vi "myRIO v1.0 Enable Encoder.vi"(8 "error in (no error)":errorcluster, 9 "Enable":bool, 10 "Channel":T1, 11 "myRIO Ref In":T2) -> (0 "error out":errorcluster, 3 "myRIO Ref Out":T2)   [LabVIEW 2021]
uses:
  <vilib>/myRIO/Common/Instrument Driver Framework/Utilities/typedefs/myRIO v1.0 Reference.ctl
  <vilib>/myRIO/Common/Instrument Driver Framework/Utilities/typedefs/Generic FPGA Reference.ctl
  <vilib>/myRIO/Common/Instrument Driver Framework/myRIO v1.0/Encoder/typedefs/Encoder Channels Enum.ctl
  <vilib>/myRIO/Common/Instrument Driver Framework/myRIO v1.0/Encoder/typedefs/Encoder Channels FPGA Reference.ctl
  <vilib>/rvi/errors/niLvFpgaAdjustHostInterfaceError.vi
  <vilib>/rvi/interface/nirviReadWriteControl/nirviReadWriteControl.xnode
  <vilib>/rvi/interface/Simulation/niFpgaSimulationCallBeginRW.vi
  NiFpgaLv.dll
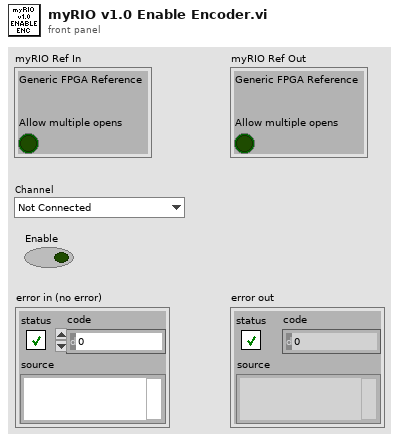
[diagram p1: front panel]
types:
  T1 = typedef "Encoder Channels Enum.ctl" = enum16{"Not Connected", "C/ENC0", "C/ENC1", "A/ENC", "A/ENC0", "A/ENC1", "A/ENC2", "A/ENC3", "A/ENC4", "A/ENC5", "A/ENC6", "A/ENC7", "A/ENC8", "A/ENC9", "B/ENC", "B/ENC0", "B/ENC1", "B/ENC2", "B/ENC3", "B/ENC4", "B/ENC5", "B/ENC6", "B/ENC7", "B/ENC8", "B/ENC9", "DIO/ENC0", "DIO/ENC1", "DIO/ENC2", "DIO/ENC3", "DIO/ENC4"}
  T2 = typedef "myRIO v1.0 Reference.ctl" = cluster{"Generic FPGA Reference":T3, "Allow multiple opens":bool}
  T3 = typedef "Generic FPGA Reference.ctl" = refnum<k20>
  T4 = typedef "Encoder Channels FPGA Reference.ctl" = refnum<k20>
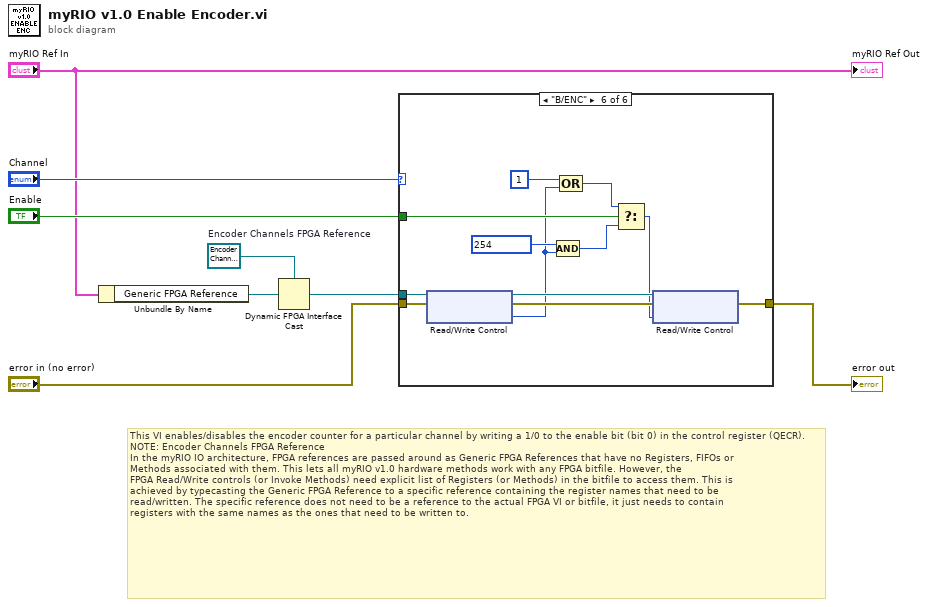
[diagram p0: block diagram]
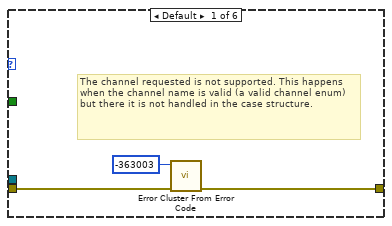
[diagram p2: hidden frame]
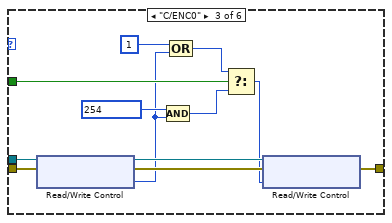
[diagram p4: hidden frame]
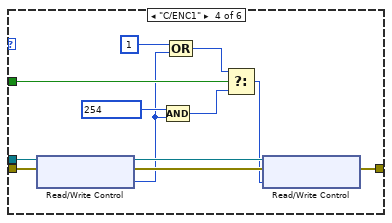
[diagram p5: hidden frame]
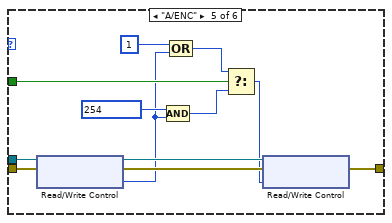
[diagram p6: hidden frame]
diagram:
  w8 = T4 refnum  # Encoder Channels FPGA Reference
  # "This VI enables/disables the encoder counter for a particular channel by writing a 1/0 to the enable bit (bit 0) in the control register (QECR).\nNOTE: Encoder Channels FPGA Reference\nIn the myRIO IO architecture, FPGA references are passed around as Generic FPGA References that have no Registers, FIFOs or\nMethods associated with them. This lets all myRIO v1.0 hardware methods work with any FPGA bitfile. However, the \nFPGA Read/Write controls (or Invoke Methods) need explicit list of Registers (or Methods) in the bitfile to access them. This is \nachieved by typecasting the Generic FPGA Reference to a specific reference containing the register names that need to be \nread/written. The specific reference does not need to be a reference to the actual FPGA VI or bitfile, it just needs to contain \nregisters with the same names as the ones that need to be written to."
  n1 = Unbundle By Name("myRIO Ref In") -> ("Generic FPGA Reference"=w2:T3)
  n2 = Dynamic FPGA Interface Cast(Session In=w8, Type=w2) -> (Session Out=w7:T4)
  n3 = case shown="\"B/ENC\"" "Channel" {
    tunnel: "error in (no error)" -> [w9 w12 w18 w30 w42 w54]
    tunnel: [w10 w12 w14 w26 w38 w50] -> w4
    tunnel: w7 -> [_ _ w19 w31 w43 w55]
    tunnel: "Enable" -> [_ _ w24 w36 w48 w60]
    frame Default {
      # "The channel requested is not supported. This happens when the channel name is valid (a valid channel enum) but there it is not handled in the case structure."
      n4 = call <vilib>:"Error Cluster From Error Code.vi"("error in (no error)"=w9, "error code (0)"=-363003) -> ("error out"=w10:errorcluster)  [unwired: 7 in]
    }
    frame "Not Connected" {
    }
    frame "C/ENC0" {
      n5 = xnode "Read/Write Control"("FPGA VI Reference In"=w19, "error in"=w18) -> ("FPGA VI Reference Out"=w17:T4, "error out"=w16:errorcluster, "ENC.C_0.CNFG"=w13:u8)
      n6 = Compound Arithmetic op=AND(u8 254, w13) -> (w23:u8)
      n7 = Compound Arithmetic op=OR(u8 1, w13) -> (w21:u8)
      n8 = Select(t=w21, s=w24, f=w23) -> (s? t:f=w15:u8)
      n9 = xnode "Read/Write Control"("FPGA VI Reference In"=w17, "error in"=w16, "ENC.C_0.CNFG"=w15) -> ("error out"=w14:errorcluster)  [unwired: 1 out]
    }
    frame "C/ENC1" {
      n10 = xnode "Read/Write Control"("FPGA VI Reference In"=w31, "error in"=w30) -> ("FPGA VI Reference Out"=w29:T4, "error out"=w28:errorcluster, "ENC.C_1.CNFG"=w25:u8)
      n11 = Compound Arithmetic op=AND(u8 254, w25) -> (w35:u8)
      n12 = Compound Arithmetic op=OR(u8 1, w25) -> (w33:u8)
      n13 = Select(t=w33, s=w36, f=w35) -> (s? t:f=w27:u8)
      n14 = xnode "Read/Write Control"("FPGA VI Reference In"=w29, "error in"=w28, "ENC.C_1.CNFG"=w27) -> ("error out"=w26:errorcluster)  [unwired: 1 out]
    }
    frame "A/ENC" {
      n15 = xnode "Read/Write Control"("FPGA VI Reference In"=w43, "error in"=w42) -> ("FPGA VI Reference Out"=w41:T4, "error out"=w40:errorcluster, "ENC.A.CNFG"=w37:u8)
      n16 = Compound Arithmetic op=AND(u8 254, w37) -> (w47:u8)
      n17 = Compound Arithmetic op=OR(u8 1, w37) -> (w45:u8)
      n18 = Select(t=w45, s=w48, f=w47) -> (s? t:f=w39:u8)
      n19 = xnode "Read/Write Control"("FPGA VI Reference In"=w41, "error in"=w40, "ENC.A.CNFG"=w39) -> ("error out"=w38:errorcluster)  [unwired: 1 out]
    }
    frame "B/ENC" {
      n20 = xnode "Read/Write Control"("FPGA VI Reference In"=w55, "error in"=w54) -> ("FPGA VI Reference Out"=w53:T4, "error out"=w52:errorcluster, "ENC.B.CNFG"=w49:u8)
      n21 = Compound Arithmetic op=AND(u8 254, w49) -> (w59:u8)
      n22 = Compound Arithmetic op=OR(u8 1, w49) -> (w57:u8)
      n23 = Select(t=w57, s=w60, f=w59) -> (s? t:f=w51:u8)
      n24 = xnode "Read/Write Control"("FPGA VI Reference In"=w53, "error in"=w52, "ENC.B.CNFG"=w51) -> ("error out"=w50:errorcluster)  [unwired: 1 out]
    }
  }
  "error out" <- w4
  "myRIO Ref Out" <- "myRIO Ref In"
